vi "Enable All Items.vi"(8 "error in":errorcluster, 11 "Data in":T1) -> (0 "error out":errorcluster, 3 "Data out":T1)   [LabVIEW 2020, in "Peek Window.lvlib"]
uses:
  Peek Window.lvlib
  Open Diagram Argument--cluster.ctl
  MHL Data Cluster.ctl
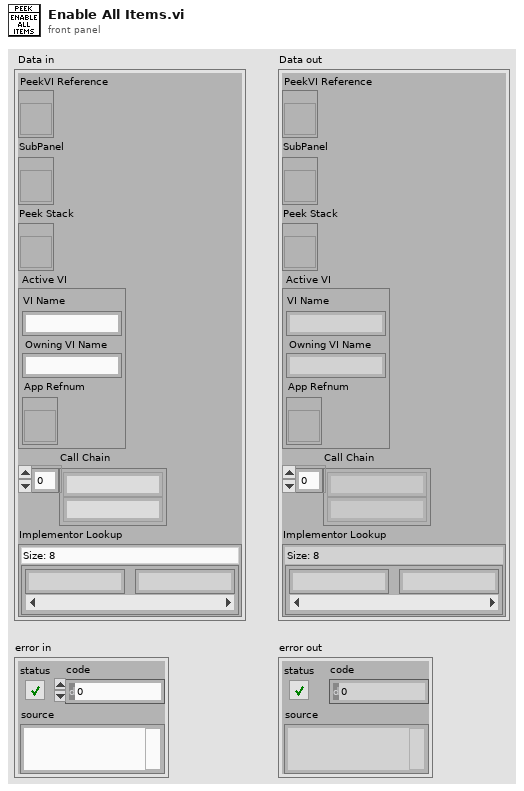
[diagram p1: front panel]
types:
  T1 = typedef "Peek Window.lvlib/MHL Data Cluster.ctl" = cluster{"PeekVI Reference":refnum<vi>, "SubPanel":refnum<vi>, "Peek Stack":refnum<vi>, "Active VI":T2, "Call Chain":string[], "Implementor Lookup":map{string, string}}
  T2 = typedef "Peek Window.lvlib/Open Diagram Argument--cluster.ctl" = cluster{"VI Name":string, "Owning VI Name":string, "App Refnum":refnum<vi>}
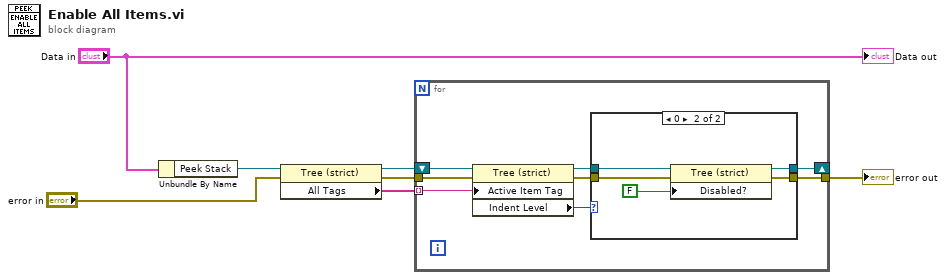
[diagram p0: block diagram]
diagram:
  n1 = Unbundle By Name("Data in") -> ("Peek Stack"=w6:refnum<vi>)
  n2 = property class="Tree (strict)"(reference=w6, error in="error in") -> (reference out=w3:refnum<vi>, error out=w2:errorcluster, "All Tags"=w4:string[])
  n3 = for {
    tunnel: w4 -> [w14] mode=indexing
    tunnel: w2 -> [w11]
    shift-right: [w9] -> _
    shift-left: w3 -> [w15]
    tunnel: [w8] -> w1
    n4 = property class="Tree (strict)"(reference=w15, error in=w11, "Active Item Tag"=w14) -> (reference out=w12:refnum<vi>, error out=w10:errorcluster, "Indent Level"=w13:i32)
    n5 = case shown="0" w13 {
      tunnel: w12 -> [w17 w22]
      tunnel: w10 -> [w16 w20]
      tunnel: [w17 w19] -> w9
      tunnel: [w16 w18] -> w8
      frame Default {
      }
      frame 0 {
        n6 = property class="Tree (strict)"(reference=w22, error in=w20, "Disabled?"=FALSE) -> (reference out=w19:refnum<vi>, error out=w18:errorcluster)
      }
    }
  }
  "error out" <- w1
  "Data out" <- "Data in"
